vi "Main.vi"(11 "Module Admin":refnum<class "Delacor_lib_QMH_Module Admin.lvclass">) -> ()   [LabVIEW 2020, in "Logging.lvlib"]
doc: "This template is based off of the Queued Message Handler design pattern and the Queued Message Handler project template that ships with LabVIEW.\n\nThe main difference is that the queue is private to this module and communication between modules is performed via Broadcast and Request events.\n\nRequest events are wrapped in public API methods and are handled in the Event Handling Loop (EHL) of this VI. Any module can register for Broadcast events sent by this module. The EHL generates messages based on user interface actions.\n\nThe Message Handling Loop (MHL) processes messages generated by the EHL, or by other messages. The messages are string values, so new messages can be added easily to the Message Cases case structure in the MHL. Each message cluster can also provide an optional value for Message Data, which is a variant that can be converted to whatever message-specific data is required.\n_____\nBased on Delacor QMH Project Template 6.0.0.89."
uses:
  Logging.lvlib
  <vilib>/Delacor/Delacor QMH/Libraries/Module Admin_class/Delacor_lib_QMH_Module Admin.lvclass
  Module Data--cluster.ctl
  Stop Argument--cluster.ctl
  <vilib>/Delacor/Delacor QMH/Libraries/Message Queue_class/Delacor_lib_QMH_Message Queue.lvclass/Delacor_lib_QMH_Message Queue.ctl
  <vilib>/Delacor/Delacor QMH/Libraries/Module Admin_class/Delacor_lib_QMH_Module Admin.lvclass/Delacor_lib_QMH_Module Admin.ctl
  Create TDMS Argument--cluster.ctl
  Write TDMS Analog Argument--cluster.ctl
  Aqcisition/Analog Signal Config.ctl
  Write TDMS Digital Argument--cluster.ctl
  Aqcisition/Digital Signal Config.ctl
  <vilib>/Utility/miscctls.llb/LVPointTypeDef.ctl
  <vilib>/Utility/sysdir.llb/System Directory Type.ctl
  <vilib>/Delacor/Delacor QMH/Libraries/Message Queue_class/Delacor_lib_QMH_Enqueue Message (Single).vi
  <vilib>/Delacor/Delacor QMH/Libraries/Module Admin_class/Delacor_lib_QMH_Get External Launch.vi
  <vilib>/Utility/error.llb/Error Cluster From Error Code.vi
  <vilib>/ErrorRing/Error Ring.xnode
  <vilib>/Delacor/Delacor QMH/Libraries/Message Queue_class/Delacor_lib_QMH_Message Queue.lvclass
panel:
  out "error out":errorcluster
  out "Status":string
types:
  T1 = typedef "Logging.lvlib/Request Events--cluster.ctl" = cluster{"Stop Module":refnum<user-event>, "Show Panel":refnum<user-event>, "Hide Panel":refnum<user-event>, "Get Module Execution Status":refnum<user-event>, "Show Diagram":refnum<user-event>, "Create TDMS":refnum<user-event>, "Write TDMS Analog":refnum<user-event>, "Write TDMS Digital":refnum<user-event>}
  T2 = typedef "Logging.lvlib/Module Data--cluster.ctl" = cluster{"Status":string}
  T3 = enum32{"invalid lock state", "Not Locked", "Locked (No Password)", "Password-protected"}
  T4 = typedef "Logging.lvlib/Stop Argument--cluster.ctl" = cluster{"Origin":string, "Exit via Stop Module Req?":bool, "Wait for Module to stop?":bool}
  T5 = typedef "Logging.lvlib/Create TDMS Argument--cluster.ctl" = cluster{"Nombre Ruta":string}
  T6 = typedef "Logging.lvlib/Write TDMS Analog Argument--cluster.ctl" = cluster{"Señal Analogica":T7, "Analog signal":dbl[]}
  T7 = typedef "Analog Signal Config.ctl" = cluster{"Canal/Canales":string, "Canal":tag, "Canales":tag[], "Frecuencia de muestreo":i32, "Numero de muestras":i32, "Tiempo de AQ":dbl}
  T8 = typedef "Logging.lvlib/Write TDMS Digital Argument--cluster.ctl" = cluster{"Señal Digital":T9, "Digital Signal":bool[]}
  T9 = typedef "Digital Signal Config.ctl" = cluster{"Puertos/Pines":string, "Puerto":tag, "Pines":tag[], "Tiempo de AQ":dbl, "Tiempo entre AQ":dbl}
  T10 = typedef "LVPointTypeDef.ctl" = cluster{"Horizontal":i16, "Vertical":i16}
  T11 = enum32{"Invalid", "Standard", "Closed", "Hidden", "Minimized", "Maximized"}
  T12 = enum16{"open", "open or create", "create or replace", "create", "open (read-only)"}
  T13 = typedef "System Directory Type.ctl" = i32
  T14 = cluster{"Canales[0]":tag, "Canales[1]":tag, "Canales[2]":tag, "Canales[3]":tag, "Canales[4]":tag, "Canales[5]":tag, "Canales[6]":tag, "Canales[7]":tag, "Canales[8]":tag}
  T15 = cluster{"Pines[0]":tag, "Pines[1]":tag, "Pines[2]":tag, "Pines[3]":tag, "Pines[4]":tag, "Pines[5]":tag, "Pines[6]":tag, "Pines[7]":tag, "Pines[8]":tag}
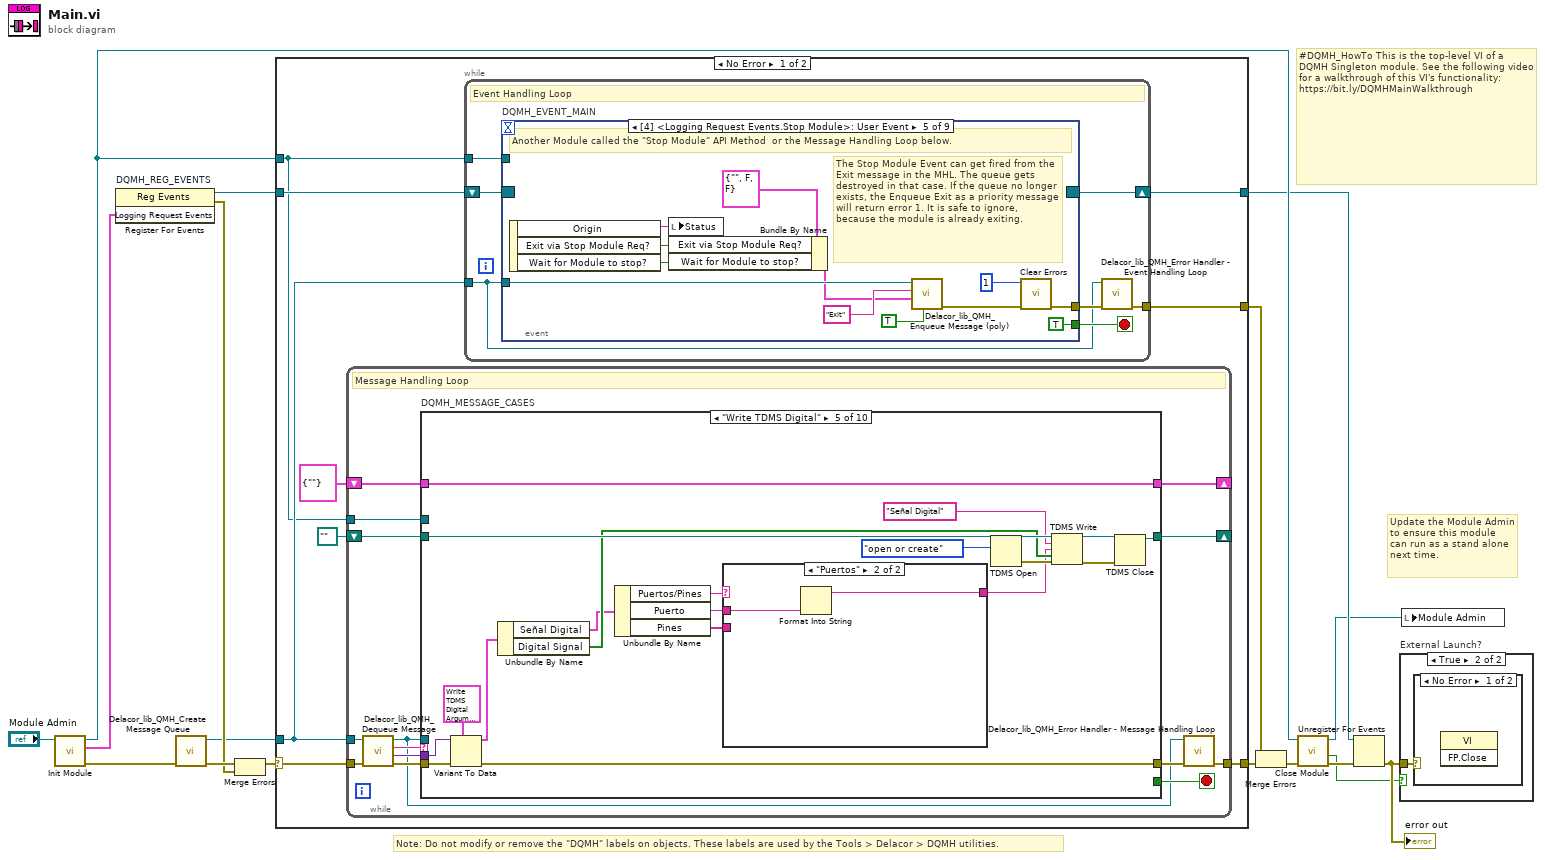
[diagram p0: block diagram]
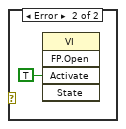
[diagram p3: hidden frame]
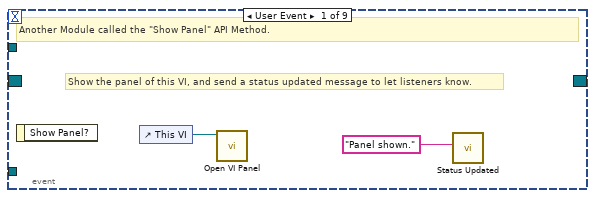
[diagram p4: hidden frame]
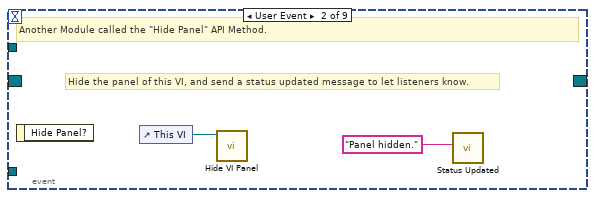
[diagram p5: hidden frame]
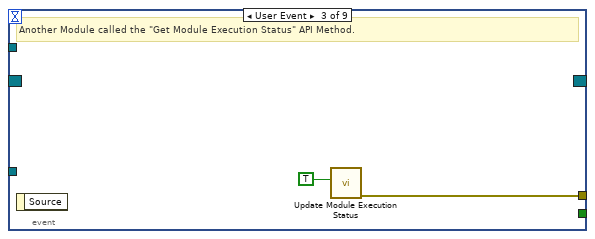
[diagram p6: hidden frame]
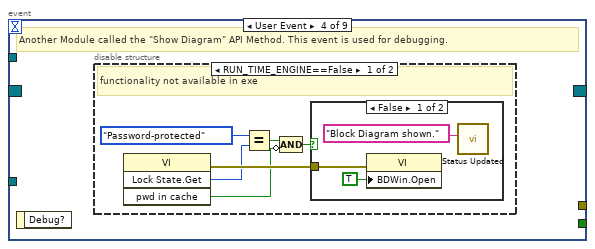
[diagram p7: hidden frame]
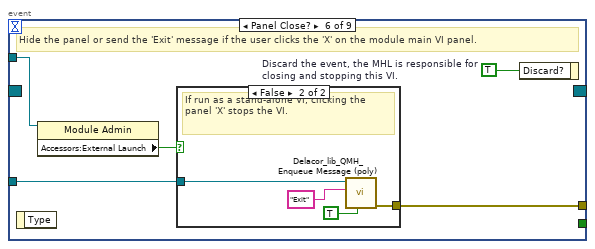
[diagram p10: hidden frame]
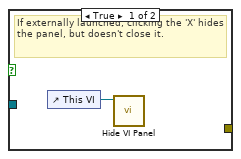
[diagram p11: hidden frame]
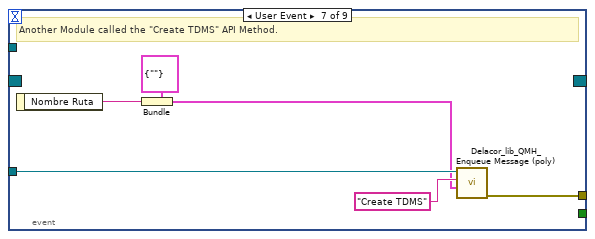
[diagram p12: hidden frame]
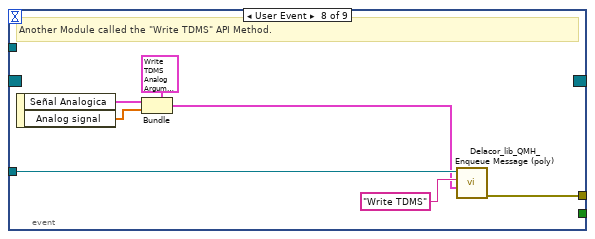
[diagram p13: hidden frame]
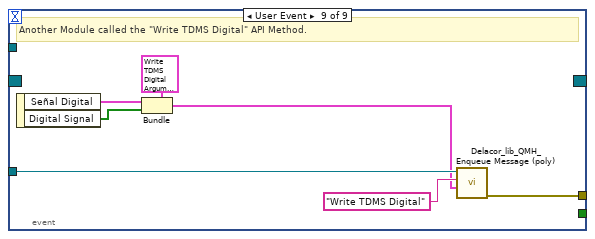
[diagram p14: hidden frame]
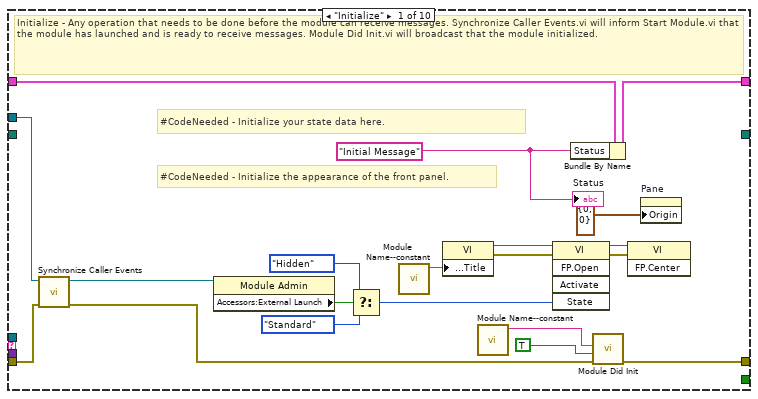
[diagram p15: hidden frame]
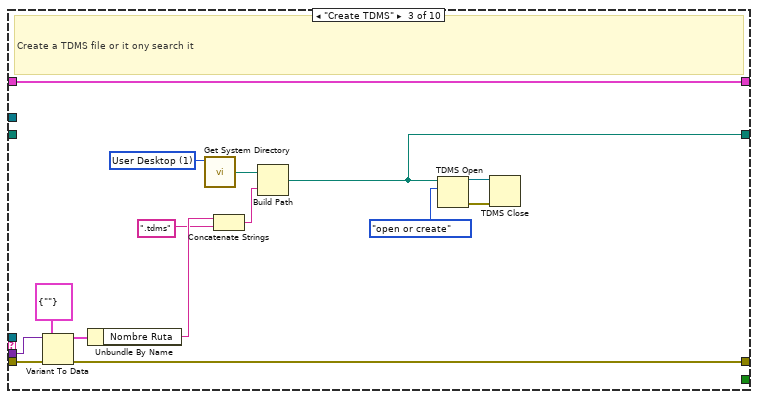
[diagram p17: hidden frame]
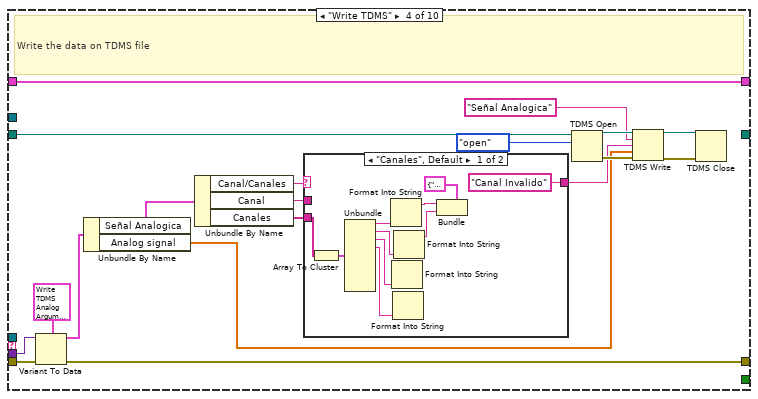
[diagram p18: hidden frame]
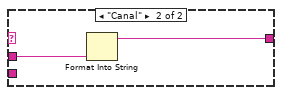
[diagram p19: hidden frame]
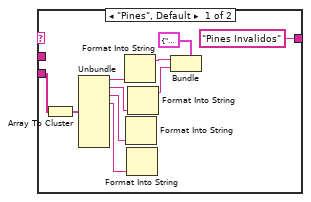
[diagram p20: hidden frame]
diagram:
  # "#DQMH_HowTo This is the top-level VI of a DQMH Singleton module. See the following video for a walkthrough of this VI's functionality: https://bit.ly/DQMHMainWalkthrough"
  # "Note: Do not modify or remove the \"DQMH\" labels on objects. These labels are used by the Tools > Delacor > DQMH utilities."
  # "Update the Module Admin to ensure this module can run as a stand alone next time."
  n1 = call "Init Module.vi"("Singleton Module Admin in"="Module Admin") -> ("error out"=w16:errorcluster, "Logging Request Events"=w5:T1, "Singleton Module Admin out"=w8:refnum<class "Delacor_lib_QMH_Module Admin.lvclass">)  [unwired: 8 in]
  n2 = register-events "DQMH_REG_EVENTS"(w5) -> (reference out=w6:refnum<event-registration>, error out=w9:errorcluster)  [unwired: 2 in]
  n3 = call <vilib>:"Delacor_lib_QMH_Create Message Queue.vi"("error in"=w16) -> ("error out"=w11:errorcluster, "Message Queue"=w4:refnum<class "Delacor_lib_QMH_Message Queue.lvclass">)  [unwired: 9 in]
  n4 = Merge Errors(w11, w9) -> (w10:errorcluster)
  n5 = case shown="No Error" w10 {
    selector: w10 -> [w24 w257]
    tunnel: [w26 w256] -> w17
    tunnel: [w23 w262] -> w7
    tunnel: w6 -> [w21 w262]
    tunnel: w4 -> [w20 w255]
    tunnel: [w25 _] -> w14
    tunnel: w8 -> [w19 w258]
    frame No Error {
      n6 = while {
        tunnel: w20 -> [w95]
        shift-right: [w99] -> _
        shift-left: T2 {"Status"=""} ("Data Cluster") -> [w100]
        tunnel: w24 -> [w103]
        tunnel: [w101] -> w26
        tunnel: w19 -> [w93]
        shift-right: [w92] -> _
        shift-left: path "" ("file path out") -> [w91]
        stop <- w98 stop-if-true
        # "Message Handling Loop"
        n7 = call-dynamic "Delacor_lib_QMH_Dequeue Message.vi"("error in"=w103, "Message Queue in"=w95) -> ("error out"=w102:errorcluster, "Message Data"=w96:variant, "Message"=w97:string, "Message Queue out"=w94:refnum<class "Delacor_lib_QMH_Message Queue.lvclass">)  [unwired: 6 in]
        n8 = case "DQMH_MESSAGE_CASES" shown="\"Write TDMS Digital\"" w97 {
          selector: w97 -> [_ _ _ _ _ _ _ _ _ w242]
          tunnel: w94 -> [_ _ _ _ _ _ _ w212 w234 _]
          tunnel: w102 -> [w122 w126 w141 w160 w192 w207 w209 w219 w240 w244]
          tunnel: [w120 w126 w139 w158 w190 w206 w209 w215 w237 w245] -> w104
          tunnel: w100 -> [w111 w125 w140 w159 w191 w205 w208 w214 w233 w243]
          tunnel: [w110 w125 w140 w159 w191 w205 w208 w214 w233 w243] -> w99
          tunnel: [_ _ _ _ _ _ _ _ w232 _] -> w98
          tunnel: w96 -> [_ _ w138 w157 w189 _ _ w213 w231 _]
          tunnel: w93 -> [w112 _ _ _ _ _ _ w211 w226 _]
          tunnel: [_ _ w130 _ w173 _ _ _ _ _] -> w92
          tunnel: w91 -> [_ _ _ w153 w177 _ _ _ _ _]
          frame "Initialize" {
            w106 = "Initial Message" ("Initial Message")
            # "#CodeNeeded - Initialize the appearance of the front panel."
            # "#CodeNeeded - Initialize your state data here."
            # "Initialize - Any operation that needs to be done before the module can receive messages. Synchronize Caller Events.vi will inform Start Module.vi that the module has launched and is ready to receive messages. Module Did Init.vi will broadcast that the module initialized."
            n9 = call "Synchronize Caller Events.vi"("error in (no error)"=w122, "Singleton Module Admin in"=w112) -> ("error out"=w121:errorcluster, "Singleton Module Admin out"=w107:refnum<class "Delacor_lib_QMH_Module Admin.lvclass">)  [unwired: 8 in]
            n10 = property class="Module Admin"(reference=w107) -> ("Accessors:External Launch"=w116:bool)  [unwired: 1 in, 2 out]
            n11 = Select(t=T11."Hidden" ("State"), s=w116, f=T11."Standard" ("State")) -> (s? t:f=w113:T11)
            n12 = call "Module Name--constant.vi"() -> ("Module Name"=w119:string)  [unwired: 11 in]
            n13 = property class="VI"("Front Panel.Title"=w119) -> (reference out=w118:refnum<vi>, error out=w124:errorcluster)  [unwired: 2 in]
            n14 = call "Module Name--constant.vi"() -> ("Module Name"=w108:string)  [unwired: 11 in]
            n15 = invoke class="VI" method="FP.Open"(reference=w118, error in=w124, "State"=w113) -> (reference out=w117:refnum<vi>, error out=w123:errorcluster)  [unwired: 2 in, 3 out]
            n16 = Bundle By Name(cluster=w111, "Status"=w106) -> (w110:T2)
            n17 = call "Module Did Init.vi"("error in (no error)"=w121, "Initialized?"=TRUE, "Origin"=w108) -> ("error out"=w120:errorcluster)  [unwired: 8 in]
            n18 = invoke class="VI" method="FP.Center"(reference=w117, error in=w123) -> ()  [unwired: 1 in, 3 out]
            n19 = property on="Pane" class="Pane"("Origin"=T10 {"Horizontal"=0, "Vertical"=0}) -> ()  [unwired: 2 in, 2 out]
            "Status" <- w106
          }
          frame "---Module Specific---" {
            # "Separator -- The following cases handle messages specific to this Module."
          }
          frame "Create TDMS" {
            w132 = T13 1 items=["User Home"=0, "User Desktop"=1, "User Documents"=2, "User Application Data"=3, "User Preferences"=4, "User Temporary"=5, "Public Documents"=6, "Public Application Data"=7, "Public Preferences"=8, "Public Cache"=13, "System Core Libraries"=9, "System Installed Libraries"=10, "Application Files"=11, "Boot Volume Root"=12] ("system directory type")
            # "Create a TDMS file or it ony search it"
            n20 = Variant To Data(error in=w141, type=T5 {"Nombre Ruta"=""} ("Create TDMS Argument"), Variant=w138) -> (data=w136:T5, error out=w139:errorcluster)
            n21 = Unbundle By Name(w136) -> ("Nombre Ruta"=w128:string)
            n22 = call <vilib>:"Get System Directory.vi"("system directory type"=w132) -> ("system directory"=w131:path)  [unwired: 10 in]
            n23 = Concatenate Strings(w128, ".tdms" ("string")) -> (w129:string)
            n24 = Build Path(base path=w131, name or relative path=w129) -> (appended path=w130:path)
            n25 = TDMS Open(10:T12."open or create" ("operation (0:open)"), 11:w130) -> (0:w133:errorcluster, 3:w134:refnum<k34>)  [unwired: 5 in]
            n26 = TDMS Close(8:w133, 11:w134) -> ()  [unwired: 2 out]
          }
          frame "Write TDMS" {
            # "Write the data on TDMS file"
            n27 = Variant To Data(error in=w160, type=T6 {"Señal Analogica"={"Canal/Canales"="", "Canal"="DAQSim1", "Canales"=[], "Frecuencia de muestreo"=1000, "Numero de muestras"=1000, "Tiempo de AQ"=0.0}, "Analog signal"=[]} ("Write TDMS Argument"), Variant=w157) -> (data=w155:T6, error out=w158:errorcluster)
            n28 = Unbundle By Name(w155) -> ("Señal Analogica"=w154:T7, "Analog signal"=w142:dbl[])
            n29 = Unbundle By Name(w154) -> ("Canal/Canales"=w144:string, "Canal"=w146:tag, "Canales"=w143:tag[])
            n30 = case shown="\"Canales\", Default" w144 {
              tunnel: w146 -> [_ w172]
              tunnel: ["Canal Invalido" w171] -> w145
              tunnel: w143 -> [w170 _]
              frame "Canales", Default {
                n31 = Array To Cluster(array=w170) -> (cluster=w169:T14)
                n32 = Unbundle(w169) -> ("Canales[0]"=w168:tag, "Canales[1]"=w167:tag, "Canales[2]"=w166:tag, "Canales[3]"=w165:tag)  [unwired: 5 out]
                n33 = Format Into String(w168) -> (resulting string=w164:string)  [unwired: 3 in, 1 out]
                n34 = Format Into String(w166) -> ()  [unwired: 3 in, 2 out]
                n35 = Format Into String(w165) -> ()  [unwired: 3 in, 2 out]
                n36 = Format Into String(w167) -> (resulting string=w163:string)  [unwired: 3 in, 1 out]
                n37 = Bundle(cluster=cluster{string, string} {"", ""}, w164, w163) -> ()  [unwired: 1 out]
              }
              frame "Canal" {
                n38 = Format Into String(w172) -> (resulting string=w171:string)  [unwired: 3 in, 1 out]
              }
            }
            n39 = TDMS Open(10:T12."open" ("operation (0:open)"), 11:w153) -> (0:w148:errorcluster, 3:w151:refnum<k34>)  [unwired: 5 in]
            n40 = TDMS Write(0:w151, 5:"Señal Analogica", 7:w145, 9:w142, 11:w148) -> (4:w150:refnum<k34>, 15:w149:errorcluster)  [unwired: 1 in, 2 out]
            n41 = TDMS Close(8:w149, 11:w150) -> ()  [unwired: 2 out]
          }
          frame "Write TDMS Digital" {
            n42 = Variant To Data(error in=w192, type=T8 {"Señal Digital"={"Puertos/Pines"="", "Puerto"="DAQSim1", "Pines"=[], "Tiempo de AQ"=0.0, "Tiempo entre AQ"=0.0}, "Digital Signal"=[]} ("Write TDMS Digital Argument"), Variant=w189) -> (data=w187:T8, error out=w190:errorcluster)
            n43 = Unbundle By Name(w187) -> ("Señal Digital"=w175:T9, "Digital Signal"=w176:bool[])
            n44 = Unbundle By Name(w175) -> ("Puertos/Pines"=w179:string, "Puerto"=w180:tag, "Pines"=w178:tag[])
            n45 = case shown="\"Puertos\"" w179 {
              tunnel: w180 -> [_ w204]
              tunnel: ["Pines Invalidos" w203] -> w174
              tunnel: w178 -> [w202 _]
              frame "Pines", Default {
                n46 = Array To Cluster(array=w202) -> (cluster=w201:T15)
                n47 = Unbundle(w201) -> ("Pines[0]"=w200:tag, "Pines[1]"=w199:tag, "Pines[2]"=w198:tag, "Pines[3]"=w197:tag)  [unwired: 5 out]
                n48 = Format Into String(w200) -> (resulting string=w196:string)  [unwired: 3 in, 1 out]
                n49 = Format Into String(w198) -> ()  [unwired: 3 in, 2 out]
                n50 = Format Into String(w197) -> ()  [unwired: 3 in, 2 out]
                n51 = Format Into String(w199) -> (resulting string=w195:string)  [unwired: 3 in, 1 out]
                n52 = Bundle(cluster=cluster{string, string} {"", ""}, w196, w195) -> ()  [unwired: 1 out]
              }
              frame "Puertos" {
                n53 = Format Into String(w204) -> (resulting string=w203:string)  [unwired: 3 in, 1 out]
              }
            }
            n54 = TDMS Open(10:T12."open or create" ("operation (0:open)"), 11:w177) -> (0:w182:errorcluster, 3:w185:refnum<k34>)  [unwired: 5 in]
            n55 = TDMS Write(0:w185, 5:"Señal Digital", 7:w174, 9:w176, 11:w182) -> (4:w184:refnum<k34>, 15:w183:errorcluster)  [unwired: 1 in, 2 out]
            n56 = TDMS Close(8:w183, 11:w184) -> (3:w173:path)  [unwired: 1 out]
          }
          frame "---Copy This Frame---" {
            # "Duplicate this frame when creating new messages.  Change this comment in the duplicated frame to describe this message."
            n57 = Merge Errors(w207) -> (w206:errorcluster)
          }
          frame "---Exit and Error Handling---" {
            # "Separator - The following cases handle errors and exit messages."
          }
          frame "Error" {
            # "#CodeRecommended - If you ever change the name of this \"Error\" message, you'll need to update the name in the Check Loop Error.vi as well."
            # "#CodeRecommended - If the module is running in standalone mode (External Launch = FALSE), this code will pop up an error dialog and call the 'Exit' message if an error occurs. Add more fine-grained error handling here."
            # "Error - Check the error message data and respond accordingly. This message is sent by the \"Error Handler\" VIs at the end of each loop in this application."
            n58 = property class="Module Admin"(reference=w211) -> ("Accessors:External Launch"=w210:bool)  [unwired: 1 in, 2 out]
            n59 = Variant To Data(error in=w219, type=errorcluster {"status"=FALSE, "code"=0, "source"=""} ("error constant"), Variant=w213) -> (data=w220:errorcluster, error out=w217:errorcluster)
            n60 = call "Error Reported.vi"("Error"=w220) -> ()  [unwired: 10 in, 1 out]
            n61 = case shown="False" w210 {
              tunnel: [w225 _] -> w216
              tunnel: w212 -> [w223 _]
              tunnel: w220 -> [w224 _]
              frame False {
                # "If the module is running standalone, then pop up an error dialog and call the \"Exit\" message."
                n62 = call <vilib>:"Simple Error Handler.vi"("error in (no error)"=w224) -> ()  [unwired: 4 in, 5 out]
                n63 = call-poly <vilib>:"Delacor_lib_QMH_Enqueue Message (poly).vi"("Priority Message? (F)"=TRUE, "Message"="Exit", "Message Queue in"=w223) -> ("error out"=w225:errorcluster)  [unwired: 7 in, 1 out]
              }
              frame True {
                # "If the module was launched externally, calling the Error Reported broadcast VI is the only action performed by the \"Error\" message. The module's caller can then process the error appropriately."
              }
            }
            n64 = Merge Errors(w217, w216) -> (w215:errorcluster)
            n65 = local write "error out"(w215) -> ()
          }
          frame "Exit" {
            w230 = 91  # 91: not all Exit messages will have an argument
            w232 = TRUE  # Stop the VI
            # "Release the message queue reference"
            # "#CodeNeeded - Add any required cleanup code here"
            # "Exit - Exit the application."
            n66 = Variant To Data(error in=w240, type=T4 {"Origin"="", "Exit via Stop Module Req?"=FALSE, "Wait for Module to stop?"=FALSE} ("Stop Argument"), Variant=w231) -> (data=w228:T4, error out=w236:errorcluster)
            n67 = call <vilib>:"Clear Errors.vi"("error in (no error)"=w236, "specific error code to clear (0: all)"=w230) -> ("error out"=w239:errorcluster)  [unwired: 4 in, 1 out]
            n68 = control-ref of="This VI"() -> (w227:refnum<vi>)
            n69 = call-dynamic "Delacor_lib_QMH_Release Message Queue.vi"("error in"=w239, "Message Queue"=w234) -> ("error out"=w238:errorcluster)  [unwired: 9 in]
            n70 = call "Handle Exit.vi"("Stop Argument"=w228, "Admin in"=w226, "VI reference"=w227) -> ("error out"=w235:errorcluster)  [unwired: 7 in, 1 out]
            n71 = Merge Errors(w238, w235) -> (w237:errorcluster)
          }
          frame Default {
            # "'Default' case only runs if there is a message that isn't defined in any of the other cases.  Output a programming error."
            n72 = call "Module Name--constant.vi"() -> ("Module Name"=w241:string)  [unwired: 11 in]
            n73 = xnode "Error Ring"("parameter 0"=w242, "parameter 1"=w241) -> ("error out"=w246:errorcluster)
            n74 = Merge Errors(w244, w246) -> (w245:errorcluster)
          }
        }
        n75 = call-dynamic "Delacor_lib_QMH_Error Handler - Message Handling Loop.vi"("error in"=w104, "Message Queue in"=w94) -> ("dup error in"=w101:errorcluster)  [unwired: 8 in, 1 out]
      }
      n76 = while {
        tunnel: w20 -> [w27]
        shift-right: [w30] -> w23
        shift-left: w21 -> [w31]
        tunnel: [w32] -> w25
        tunnel: w19 -> [w28]
        stop <- w29 stop-if-true
        # "Event Handling Loop"
        n77 = event "DQMH_EVENT_MAIN" shown="[4] <Logging Request Events.Stop Module>: User Event" {
          selector: w31 -> [_ _ _ _ _ _ _ _ _]
          dyn-events: [_ _ _ _ _ _ _ _ _] -> w30
          timeout: _ -> [_ _ _ _ _ _ _ _ _]
          tunnel: [_ _ _ _ TRUE ("Discard?") _ _ _ _] -> w29
          tunnel: w27 -> [_ _ _ _ w56 w63 w76 w83 w90]
          tunnel: [_ _ w39 _ w59 w65 w71 w77 w84] -> w33
          tunnel: w28 -> [_ _ _ _ _ w62 _ _ _]
          event User Event {
            # "Show the panel of this VI, and send a status updated message to let listeners know."
            # "Another Module called the \"Show Panel\" API Method."
            n78 = event-data() -> ()  [unwired: 1 in, 1 out]
            n79 = control-ref of="This VI"() -> (w35:refnum<vi>)
            n80 = call "Open VI Panel.vi"("VI"=w35) -> ()  [unwired: 10 in, 1 out]
            n81 = call "Status Updated.vi"("Status"="Panel shown." ("format string")) -> ()  [unwired: 10 in, 1 out]
          }
          event User Event {
            # "Hide the panel of this VI, and send a status updated message to let listeners know."
            # "Another Module called the \"Hide Panel\" API Method."
            n82 = event-data() -> ()  [unwired: 1 in, 1 out]
            n83 = control-ref of="This VI"() -> (w37:refnum<vi>)
            n84 = call "Hide VI Panel.vi"("VI"=w37) -> ()  [unwired: 10 in, 1 out]
            n85 = call "Status Updated.vi"("Status"="Panel hidden." ("format string")) -> ()  [unwired: 10 in, 1 out]
          }
          event User Event {
            # "Another Module called the \"Get Module Execution Status\" API Method."
            n86 = event-data() -> ()  [unwired: 1 in, 1 out]
            n87 = call "Update Module Execution Status.vi"("Running?"=TRUE) -> ("error out"=w39:errorcluster)  [unwired: 10 in]
          }
          event User Event {
            # "Another Module called the \"Show Diagram\" API Method. This event is used for debugging."
            n88 = event-data() -> ()  [unwired: 1 in, 1 out]
            n89 = disable-structure shown="RUN_TIME_ENGINE==False" {
              frame condition #0 (active) {
                # "functionality not available in exe"
                n90 = invoke class="VI" method="Lock State.Get"() -> (error out=w45:errorcluster, "Get Lock State"=w44:T3, "pwd in cache"=w41:bool)  [unwired: 4 in, 1 out]
                n91 = Equal?(x=T3."Password-protected", y=w44) -> (x = y?=w42:bool)
                n92 = Compound Arithmetic op=AND(w42, invert w41) -> (w40:bool)
                n93 = case shown="False" w40 {
                  tunnel: w45 -> [w48 _]
                  frame False {
                    n94 = property class="VI"(error in=w48, "BDWin.Open"=TRUE ("Block Diagram Window:Open")) -> ()  [unwired: 1 in, 2 out]
                    n95 = call "Status Updated.vi"("Status"="Block Diagram shown." ("format string")) -> ()  [unwired: 10 in, 1 out]
                  }
                  frame True {
                    # "Password-protected VI, and the password is not in the cache. Do not show the diagram."
                  }
                }
              }
              frame condition #1 {
              }
            }
          }
          event User Event {
            # "The Stop Module Event can get fired from the Exit message in the MHL. The queue gets destroyed in that case. If the queue no longer exists, the Enqueue Exit as a priority message will return error 1. It is safe to ignore, because the module is already exiting."
            # "Another Module called the \"Stop Module\" API Method  or the Message Handling Loop below."
            n96 = event-data() -> ("Origin"=w55:string, "Exit via Stop Module Req?"=w51:bool, "Wait for Module to stop?"=w50:bool)  [unwired: 1 in]
            n97 = local write "Status"(w55) -> ()
            n98 = Bundle By Name(cluster=T4 {"Origin"="", "Exit via Stop Module Req?"=FALSE, "Wait for Module to stop?"=FALSE} ("Stop Argument"), "Exit via Stop Module Req?"=w51, "Wait for Module to stop?"=w50) -> (w49:T4)
            n99 = call-poly <vilib>:"Delacor_lib_QMH_Enqueue Message (poly).vi"("Priority Message? (F)"=TRUE, "Message Data"=w49, "Message"="Exit", "Message Queue in"=w56) -> ("error out"=w60:errorcluster)  [unwired: 6 in, 1 out]
            n100 = call <vilib>:"Clear Errors.vi"("error in (no error)"=w60, "specific error code to clear (0: all)"=1) -> ("error out"=w59:errorcluster)  [unwired: 4 in, 1 out]
          }
          event Panel Close? {
            w64 = TRUE  # Discard the event, the MHL is responsible for closing and stopping this VI.
            # "Hide the panel or send the 'Exit' message if the user clicks the 'X' on the module main VI panel."
            n101 = event-data() -> ()  [unwired: 1 in, 1 out]
            n102 = property class="Module Admin"(reference=w62) -> ("Accessors:External Launch"=w61:bool)  [unwired: 1 in, 2 out]
            n103 = case shown="False" w61 {
              tunnel: w63 -> [_ w69]
              tunnel: [_ w70] -> w65
              frame True {
                # "If externally launched, clicking the 'X' hides the panel, but doesn't close it."
                n104 = control-ref of="This VI"() -> (w66:refnum<vi>)
                n105 = call "Hide VI Panel.vi"("VI"=w66) -> ()  [unwired: 10 in, 1 out]
              }
              frame False {
                # "If run as a stand-alone VI, clicking the panel 'X' stops the VI."
                n106 = call-poly <vilib>:"Delacor_lib_QMH_Enqueue Message (poly).vi"("Priority Message? (F)"=TRUE, "Message"="Exit", "Message Queue in"=w69) -> ("error out"=w70:errorcluster)  [unwired: 7 in, 1 out]
              }
            }
            n107 = event-data("Discard?"=w64) -> ()  [unwired: 1 in, 1 out]
          }
          event User Event {
            # "Another Module called the \"Create TDMS\" API Method."
            n108 = event-data() -> ("Nombre Ruta"=w72:string)  [unwired: 1 in]
            n109 = Bundle(cluster=T5 {"Nombre Ruta"=""} ("Create TDMS Argument"), "Nombre Ruta"=w72) -> (w73:T5)
            n110 = call-poly <vilib>:"Delacor_lib_QMH_Enqueue Message (poly).vi"("Message Data"=w73, "Message"="Create TDMS", "Message Queue in"=w76) -> ("error out"=w71:errorcluster)  [unwired: 7 in, 1 out]
          }
          event User Event {
            # "Another Module called the \"Write TDMS\" API Method."
            n111 = event-data() -> ("Señal Analogica"=w79:T7, "Analog signal"=w78:dbl[])  [unwired: 1 in]
            n112 = Bundle(cluster=T6 {"Señal Analogica"={"Canal/Canales"="", "Canal"="DAQSim1", "Canales"=[], "Frecuencia de muestreo"=1000, "Numero de muestras"=1000, "Tiempo de AQ"=0.0}, "Analog signal"=[]} ("Write TDMS Argument"), "Señal Analogica"=w79, "Analog signal"=w78) -> (w80:T6)
            n113 = call-poly <vilib>:"Delacor_lib_QMH_Enqueue Message (poly).vi"("Message Data"=w80, "Message"="Write TDMS", "Message Queue in"=w83) -> ("error out"=w77:errorcluster)  [unwired: 7 in, 1 out]
          }
          event User Event {
            # "Another Module called the \"Write TDMS Digital\" API Method."
            n114 = event-data() -> ("Señal Digital"=w86:T9, "Digital Signal"=w85:bool[])  [unwired: 1 in]
            n115 = Bundle(cluster=T8 {"Señal Digital"={"Puertos/Pines"="", "Puerto"="DAQSim1", "Pines"=[], "Tiempo de AQ"=0.0, "Tiempo entre AQ"=0.0}, "Digital Signal"=[]} ("Write TDMS Digital Argument"), "Señal Digital"=w86, "Digital Signal"=w85) -> (w87:T8)
            n116 = call-poly <vilib>:"Delacor_lib_QMH_Enqueue Message (poly).vi"("Message Data"=w87, "Message"="Write TDMS Digital", "Message Queue in"=w90) -> ("error out"=w84:errorcluster)  [unwired: 7 in, 1 out]
          }
        }
        n117 = call-dynamic "Delacor_lib_QMH_Error Handler - Event Handling Loop.vi"("error in"=w33, "Message Queue in"=w27) -> ("dup error in"=w32:errorcluster)  [unwired: 8 in, 1 out]
      }
    }
    frame Error {
      # "Synchronize Caller Events.vi will inform Start Module.vi that the module has launched and will let the code calling Start Module.vi register for broadcasts and would permit the caller receive the broadcast that an error occurred at launch time."
      n118 = call-dynamic "Delacor_lib_QMH_Release Message Queue.vi"("error in"=w257, "Message Queue"=w255) -> ("error out"=w256:errorcluster)  [unwired: 9 in]
      n119 = call "Synchronize Caller Events.vi"("Singleton Module Admin in"=w258) -> ("error out"=w263:errorcluster)  [unwired: 9 in, 1 out]
      n120 = call "Module Name--constant.vi"() -> ("Module Name"=w261:string)  [unwired: 11 in]
      n121 = Format Into String(format string="An error occurred during initialization. %s is no longer running.", w261) -> (resulting string=w259:string)  [unwired: 2 in, 1 out]
      n122 = Merge Errors(w256, w263) -> (w264:errorcluster)
      n123 = call "Error Reported.vi"("Additional Information"=w259, "Error"=w264) -> ()  [unwired: 9 in, 1 out]
    }
  }
  n124 = Merge Errors(w14, w17) -> (w13:errorcluster)
  n125 = call "Close Module.vi"("error in (no error)"=w13, "Module Admin in"=w8) -> ("error out"=w15:errorcluster, "External Launch"=w1:bool, "Module Admin out"=w2:refnum<class "Delacor_lib_QMH_Module Admin.lvclass">)  [unwired: 7 in]
  n126 = Unregister For Events(event registration refnum=w7, error in=w15) -> (error out=w12:errorcluster)
  "error out" <- w12
  n127 = case "External Launch?" shown="True" w1 {
    tunnel: w12 -> [_ w265]
    frame False {
    }
    frame True {
      n128 = case shown="No Error" w265 {
        frame No Error {
          n129 = invoke class="VI" method="FP.Close"() -> ()  [unwired: 3 in, 3 out]
        }
        frame Error {
          n130 = invoke class="VI" method="FP.Open"("Activate"=TRUE ("Activate?")) -> ()  [unwired: 4 in, 5 out]
        }
      }
    }
  }
  n131 = local write "Module Admin"(w2) -> ()
